vi "Write serialCommunicator.vi"(10 "serialCommunicator":refnum<class "SerialCommunicator.lvclass">, 11 "TemperatureSensor in":refnum<class "TemperatureSensor.lvclass">) -> (3 "TemperatureSensor out":refnum<class "TemperatureSensor.lvclass">)   [LabVIEW 2013, in "TemperatureSensor.lvlib" / "TemperatureSensor.lvclass"]
uses:
  <userlib>/Common/Devices/TemperatureSensor/TemperatureSensor/TemperatureSensor.lvclass
  <userlib>/Common/SerialProtocols/SerialCommunicator/SerialCommunicator.lvclass
  <userlib>/Common/Devices/TemperatureSensor/TemperatureSensor/TemperatureSensor.lvclass/TemperatureSensor.ctl
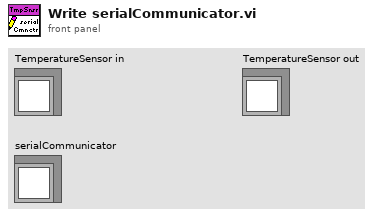
[diagram p1: front panel]
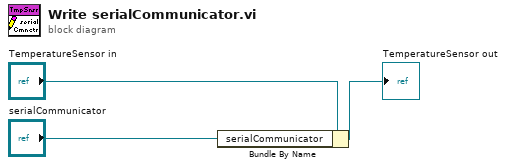
[diagram p0: block diagram]
diagram:
  n1 = Bundle By Name(cluster="TemperatureSensor in", "serialCommunicator"="serialCommunicator") -> (→"TemperatureSensor out":refnum<class "TemperatureSensor.lvclass">)
